vi "Read Query.vi"(8 "error in (no error)":errorcluster, 11 "URI in":refnum<class "URI.lvclass">) -> (0 "error out":errorcluster, 2 "Query":cluster{"argument":string, "value":string}[](array[cluster]), 3 "URI out":refnum<class "URI.lvclass">)   [LabVIEW 2013, in "openURI.lvlib" / "URI.lvclass"]
uses:
  URI.lvclass
  URI.lvclass/URI.ctl
  components/query/URI-Component.Query.lvclass/URI-Component.Query.ctl
  components/query/URI-Component.Query.lvclass
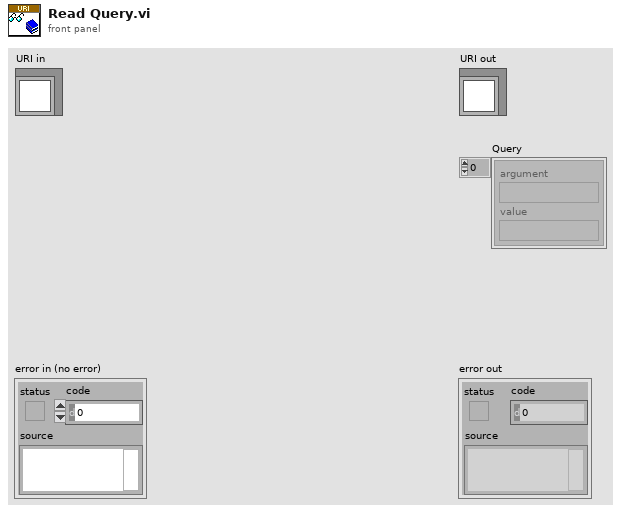
[diagram p1: front panel]
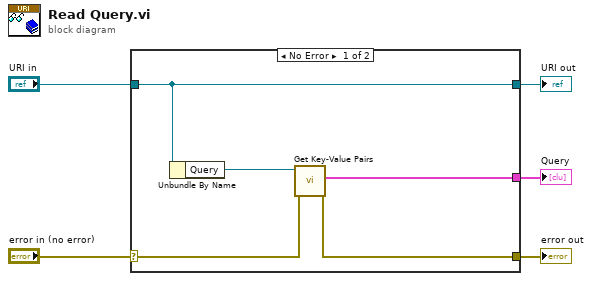
[diagram p0: block diagram]
diagram:
  n1 = case shown="No Error" "error in (no error)" {
    selector: "error in (no error)" -> [w7 w11]
    tunnel: [w6 w11] -> w4
    tunnel: [w10 w12] -> w2
    tunnel: "URI in" -> [w10 w12]
    tunnel: [w8 _] -> w1
    frame No Error {
      n2 = Unbundle By Name(w10) -> ("Query"=w9:refnum<class "URI-Component.Query.lvclass">)
      n3 = call "Get Key-Value Pairs.vi"("error in (no error)"=w7, "URI-Component.Query in"=w9) -> ("error out"=w6:errorcluster, "Query"=w8:cluster{"argument":string, "value":string}[])  [unwired: 7 in, 1 out]
    }
    frame Error {
    }
  }
  "error out" <- w4
  "URI out" <- w2
  "Query" <- w1
